vi "Wait for UEGO HW Settling.vi"(6 "HW Settling Time Ticks":u32, 7 "Starting Index":i32, 8 "Current Tick Count in":u32[](array[numeric]), 9 "Prev States":bool[](array[boolean]), 10 "Current Values":dbl[](array[numeric]), 11 "Previous Values":dbl[](array[numeric])) -> (0 "Current Tick Count out":u32[](array[numeric]), 1 "Current States":bool[](array[boolean]), 2 "New State":bool[](array[boolean]), 3 "Update State?":bool)   [LabVIEW 2014, in "SLSC configuration Engine.lvlib"]
uses:
  SLSC configuration Engine.lvlib
  Shared/Constants.vi
  Shared/SLSC configuration Shared.lvlib
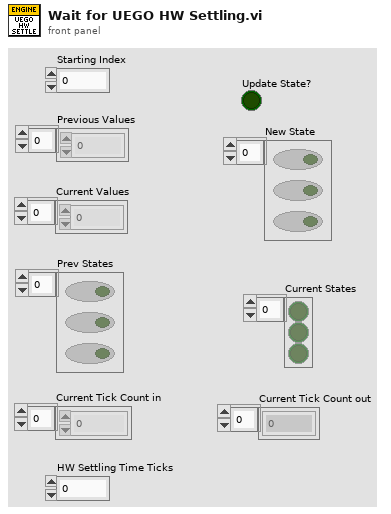
[diagram p1: front panel]
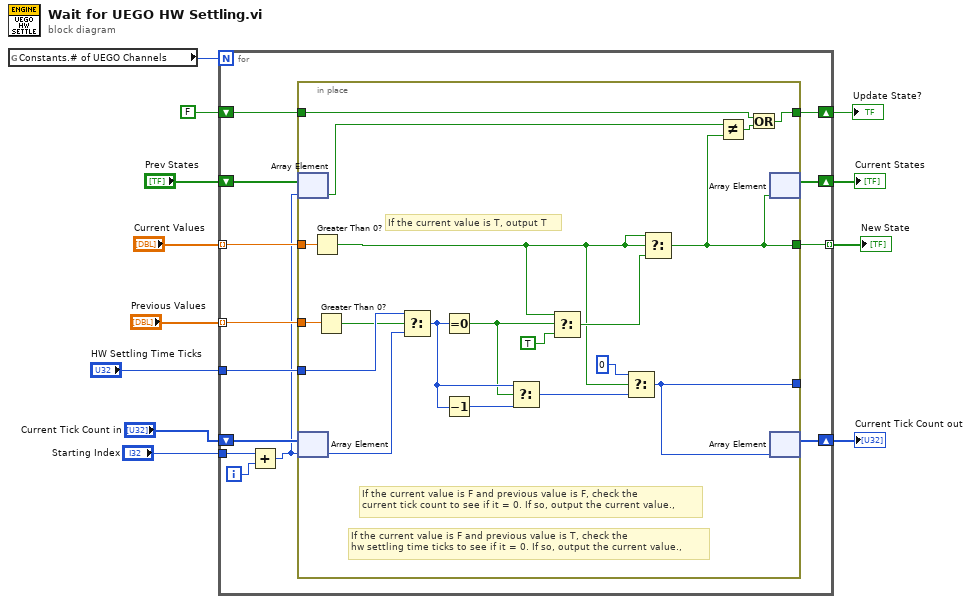
[diagram p0: block diagram]
diagram:
  n1 = global read "Constants.vi" "Constants.# of UEGO Channels"() -> (w6:u8)
  n2 = for {
    N: w6 -> [_]
    tunnel: "Current Values" -> [w25] mode=indexing
    tunnel: [w23] -> w10 mode=indexing
    tunnel: "HW Settling Time Ticks" -> [w22]
    tunnel: "Previous Values" -> [w24] mode=indexing
    shift-right: [w20] -> w5
    shift-left: "Current Tick Count in" -> [w21]
    tunnel: "Starting Index" -> [w18]
    shift-right: [w13] -> w3
    shift-left: FALSE -> [w14]
    shift-right: [w15] -> w1
    shift-left: "Prev States" -> [w17]
    i -> [w19]
    n3 = Add(x=w18, y=w19) -> (x+y=w16:i32)
    n4 = in-place {
      in-place-border: w25 -> [w44]
      in-place-border: w24 -> [w43]
      in-place-border: [w30] -> w23
      in-place-border: w22 -> [w42]
      in-place-border: [w35] -> _
      in-place-border: w14 -> [w28]
      in-place-border: [w27] -> w13
      # "If the current value is F and previous value is T, check the\nhw settling time ticks to see if it = 0. If so, output the current value.,"
      # "If the current value is F and previous value is F, check the\ncurrent tick count to see if it = 0. If so, output the current value.,"
      # "If the current value is T, output T"
      n5 = in-place-array #1(w17, w16) -> (w31:bool)
      n6 = in-place-array #2(w21, w16) -> (w34:u32)
      n7 = Greater Than 0?(x=w44) -> (x > 0?=w26:bool)
      n8 = Greater Than 0?(x=w43) -> (x > 0?=w33:bool)
      n9 = Select(t=w42, s=w33, f=w34) -> (s? t:f=w39:u32)
      n10 = Equal To 0?(x=w39) -> (x = 0?=w32:bool)
      n11 = Decrement(x=w39) -> (x-1=w38:u32)
      n12 = Select(t=w39, s=w32, f=w38) -> (s? t:f=w36:u32)
      n13 = Select(t=w26, s=w32, f=TRUE) -> (s? t:f=w41:bool)
      n14 = Select(t=u32 0 ("s? t:f"), s=w26, f=w36) -> (s? t:f=w35:u32)
      n15 = Select(t=w26, s=w26, f=w41) -> (s? t:f=w30:bool)
      n16 = Not Equal?(x=w31, y=w30) -> (x != y?=w29:bool)
      n17 = Or(x=w28, y=w29) -> (x .or. y?=w27:bool)
      n18 = in-place-array #1(w30) -> (w15:bool[])  [unwired: 1 out]
      n19 = in-place-array #2(w35) -> (w20:u32[])  [unwired: 1 out]
    }
  }
  "New State" <- w10
  "Current Tick Count out" <- w5
  "Update State?" <- w3
  "Current States" <- w1
